vi "rad_Check IF LinuxRT.vi"(11 "Product Name":string) -> (1 "Target is 906x?":bool, 2 "Target is 903x?":bool, 3 "Target is LinuxRT?":bool)   [LabVIEW 2016]
panel:
  out "Model":string
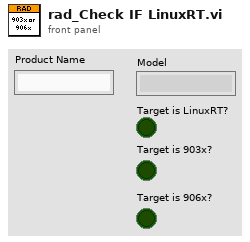
[diagram p1: front panel]
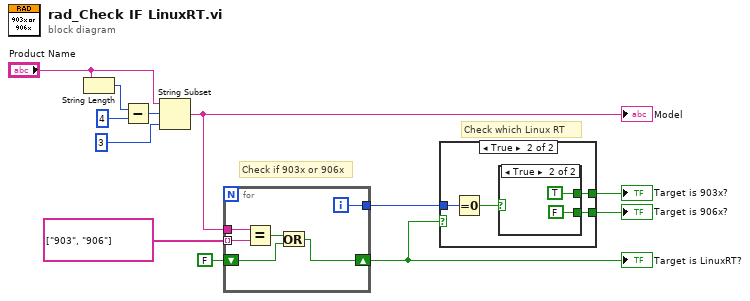
[diagram p0: block diagram]
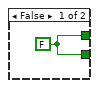
[diagram p2: hidden frame]
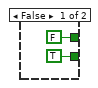
[diagram p3: hidden frame]
diagram:
  # "Check if 903x or 906x"
  # "Check which Linux RT"
  n1 = String Length(string="Product Name") -> (length=w11:i32)
  n2 = Subtract(x=w11, y=4) -> (x-y=w12:i32)
  n3 = String Subset(string="Product Name", offset (0)=w12, length (rest)=3 ("length (rest)")) -> (substring=w7:string)
  "Model" <- w7
  n4 = for {
    tunnel: string[] ["903", "906"] -> [w17] mode=indexing
    tunnel: w7 -> [w18]
    shift-right: [w14] -> w5
    shift-left: FALSE -> [w15]
    tunnel: [w13] -> w4
    i -> [w13]
    n5 = Equal?(x=w18, y=w17) -> (x = y?=w16:bool)
    n6 = Or(x=w16, y=w15) -> (x .or. y?=w14:bool)
  }
  "Target is LinuxRT?" <- w5
  n7 = case shown="True" w5 {
    tunnel: w4 -> [_ w23]
    tunnel: [w19 w21] -> w3
    tunnel: [w19 w20] -> w2
    frame False {
      w19 = FALSE
    }
    frame True {
      n8 = Equal To 0?(x=w23) -> (x = 0?=w22:bool)
      n9 = case shown="True" w22 {
        tunnel: [FALSE TRUE] -> w21
        tunnel: [TRUE FALSE] -> w20
        frame False {
        }
        frame True {
        }
      }
    }
  }
  "Target is 903x?" <- w3
  "Target is 906x?" <- w2
